vi "Write Limit Volt.vi"(8 "error in":errorcluster, 10 "OverVoltage_Protect":dbl, 11 "36234A in":refnum<class "36234A.lvclass">) -> (0 "error out":errorcluster, 3 "36234A out":refnum<class "36234A.lvclass">)   [LabVIEW 2019, in "36234A.lvlib" / "36234A.lvclass"]
uses:
  Library/36234A.lvclass
  C:/Users/Public/Documents/Development/builds/Instruments/PowerSupply.lvlibp/Library/PowerSupply.lvclass
  Library/36234A.lvclass/36234A.ctl
  builds/Instruments/PowerSupply.lvlibp/Accessors/Read Active Channel.vi
  builds/Instruments/PowerSupply.lvlibp/Library/PowerSupply.lvclass
  <instrlib>/Keysight E36000 Series/Keysight E36000 Series.lvlib
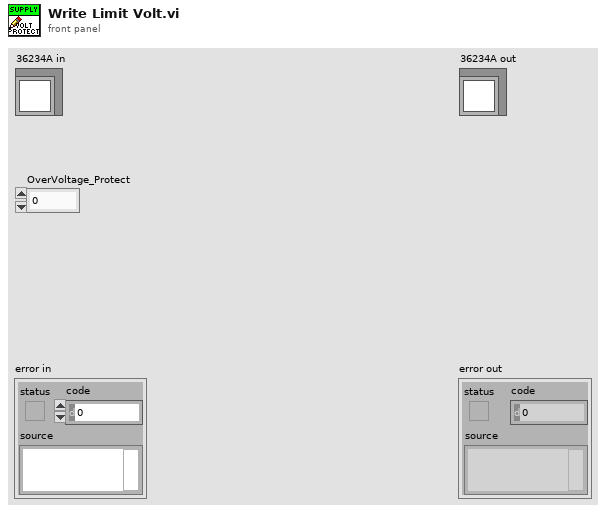
[diagram p1: front panel]
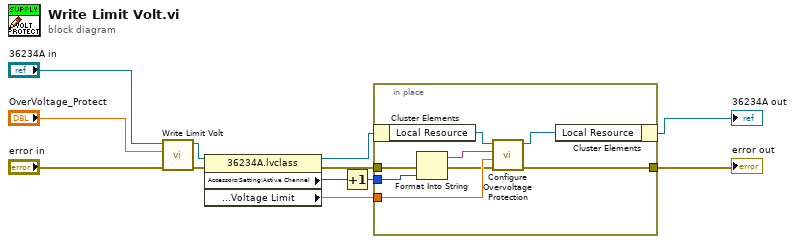
[diagram p0: block diagram]
diagram:
  n1 = call-parent "Write Limit Volt.vi"("error in"="error in", "OverVoltage_Protect"="OverVoltage_Protect", "PowerSupply in"="36234A in") -> ("error out"=w9:errorcluster, "PowerSupply out"=w5:refnum<class "36234A.lvclass">)  [unwired: 7 in]
  n2 = property class="36234A.lvclass"(reference=w5, error in=w9) -> (reference out=w4:refnum<class "36234A.lvclass">, error out=w6:errorcluster, "Accessors:Setting:Active Channel"=w3:u32, "Accessors:Setting:Protection:Voltage Limit"=w1:dbl)
  n3 = Increment(x=w3) -> (x+1=w2:u32)
  n4 = in-place {
    in-place-border: w6 -> [w14]
    in-place-border: [w18] -> w8
    in-place-border: w2 -> [w17]
    in-place-border: w1 -> [w15]
    n5 = in-place-cluster #1(w4) -> ("Local Resource"=w20:refnum<visa-resource-name>)
    n6 = Format Into String(error in=w14, w17) -> (resulting string=w16:string, error out=w13:errorcluster)  [unwired: 2 in]
    n7 = call <instrlib>:"Configure Overvoltage Protection.vi"("error in (no error)"=w13, "Voltage Limit (30.9 V)"=w15, "Channel (1)"=w16, "VISA resource name"=w20) -> ("error out"=w18:errorcluster, "VISA resource name out"=w19:refnum<visa-resource-name>)  [unwired: 6 in]
    n8 = in-place-cluster #1("Local Resource"=w19) -> (→"36234A out":refnum<class "36234A.lvclass">)
  }
  "error out" <- w8
